vi "SimpleExample_MCA_Program.vi"() -> ()   [LabVIEW 2014]
uses:
  Typedef_MCAControl.ctl
panel:
  in  "TAC Settings":cluster{"Full Scale (ns)":dbl, "# bins":i32}={"Full Scale (ns)"=1000.0, "# bins"=1000} {"# bins" min=1 max=65535 step=1; "Full Scale (ns)" format="%0.2f"}
  in  "Stop Button":bool
  out "Coincidence Signal":cluster{"Axis":dbl[], i32[]}(graph)
  out "Total Time (s)":dbl
  out "Delta Time (s)":dbl
  out "error out":errorcluster
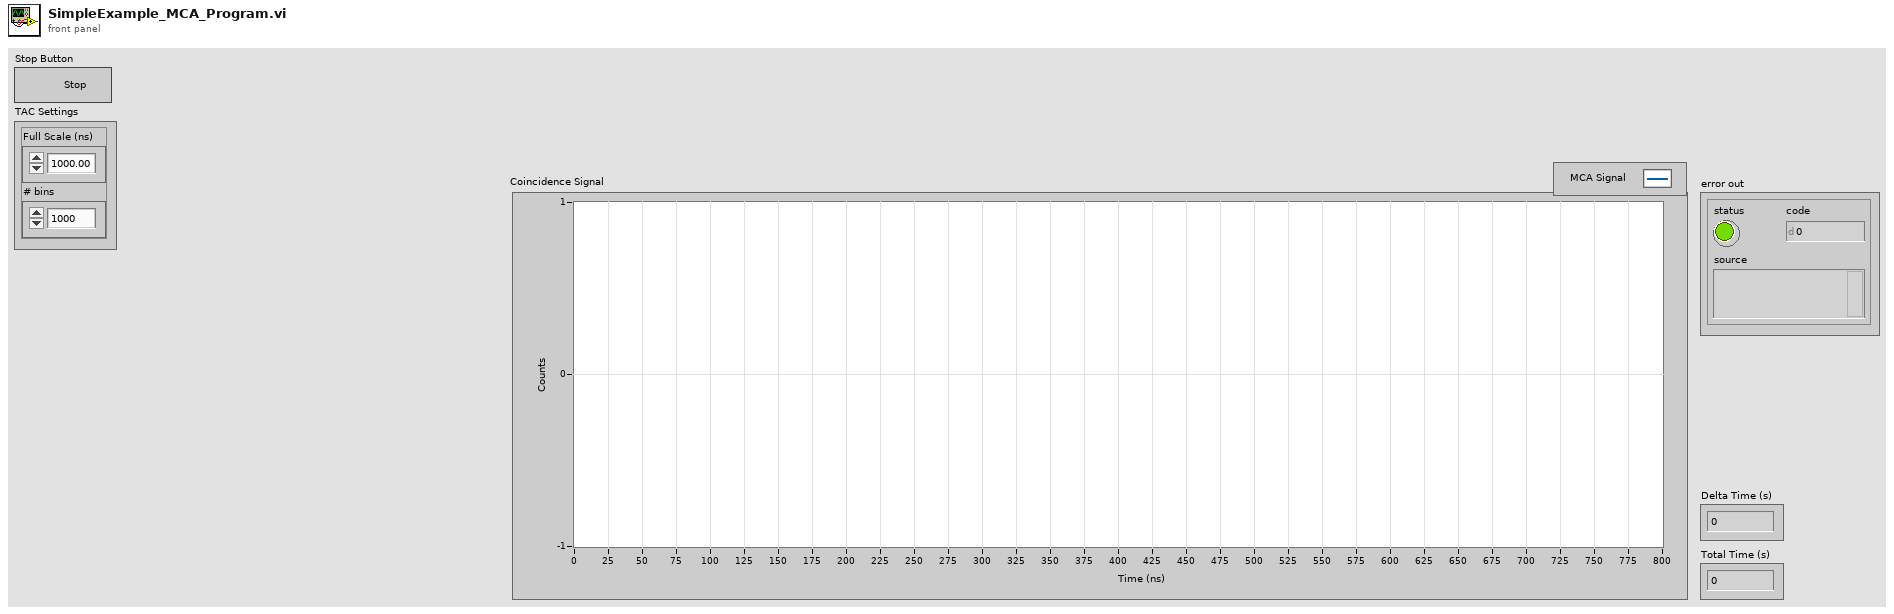
[diagram p1: front panel]
types:
  T1 = typedef "Typedef_MCAControl.ctl" = enum16{"Start", "Check", "Pause", "Unpause", "Update Settings", "Reset", "Stop"}
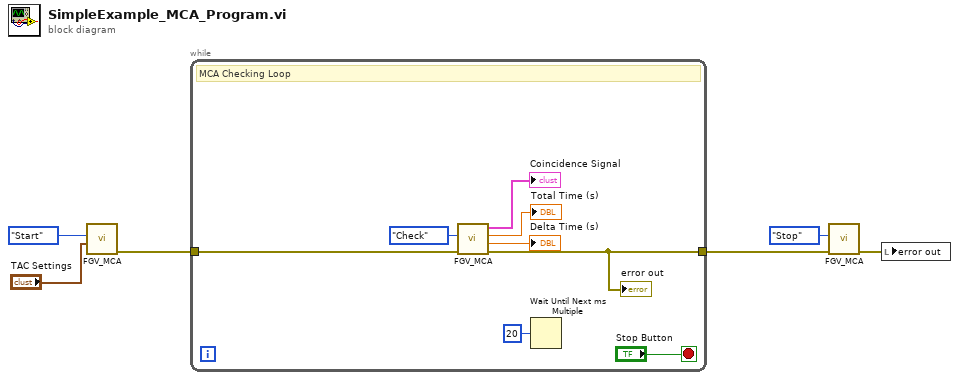
[diagram p0: block diagram]
diagram:
  n1 = call "FGV_MCA.vi"("TAC Settings"="TAC Settings", "MCA Action"=Typedef_MCAControl."Start") -> ("error out"=w6:errorcluster)  [unwired: 5 in, 4 out]
  n2 = while {
    tunnel: w6 -> [w13]
    tunnel: [w12] -> w5
    stop <- "Stop Button" stop-if-true
    # "MCA Checking Loop"
    n3 = call "FGV_MCA.vi"("Error In"=w13, "MCA Action"=Typedef_MCAControl."Check") -> ("error out"=w12:errorcluster, "Delta Time (s)"=→"Delta Time (s)":dbl, "Total Time (s)"=→"Total Time (s)":dbl, "Coincidence Signal"=→"Coincidence Signal":cluster{"Axis":dbl[], i32[]})  [unwired: 5 in, 1 out]
    "error out" <- w12
    n4 = Wait Until Next ms Multiple(millisecond multiple=u32 20) -> ()  [unwired: 1 out]
  }
  n5 = call "FGV_MCA.vi"("Error In"=w5, "MCA Action"=Typedef_MCAControl."Stop") -> ("error out"=w2:errorcluster)  [unwired: 5 in, 4 out]
  n6 = local write "error out"(w2) -> ()
